vi "SUB-Excel-Function-SLOPE.vi"(10 "Y":dbl[](array[numeric]), 11 "X":dbl[](array[numeric])) -> (1 "offset":dbl, 2 "intercept":dbl format="%#.6g", 3 "slope":dbl format="%#.6g")   [LabVIEW 2015]
uses:
  <vilib>/Analysis/baseanly.llb/Mean (DBL).vi
  <vilib>/Analysis/NI_AALBase.lvlib
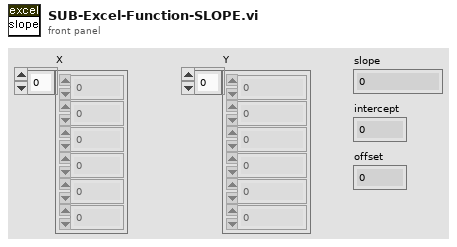
[diagram p1: front panel]
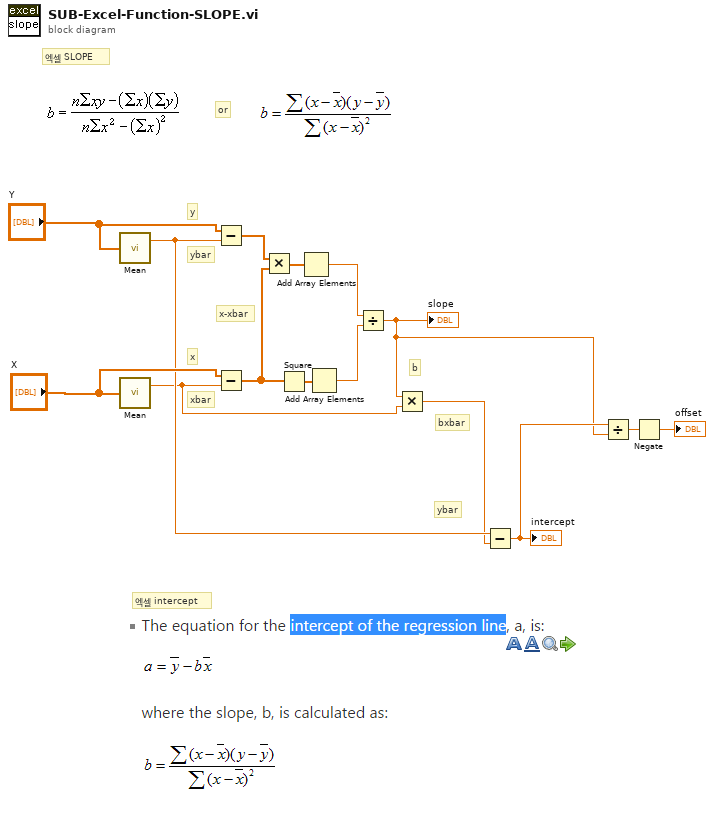
[diagram p0: block diagram]
diagram:
  # "bxbar"
  # "b"
  # "ybar"
  # "엑셀 intercept"
  # "x-xbar"
  # "y"
  # "ybar"
  # "x"
  # "xbar"
  # "or"
  # "엑셀 SLOPE"
  n1 = call-poly <vilib>:"Mean.vi"("X"="Y") -> ("mean"=w7:dbl)  [unwired: 1 out]
  n2 = call-poly <vilib>:"Mean.vi"("X"="X") -> ("mean"=w6:dbl)  [unwired: 1 out]
  n3 = Subtract(x="Y", y=w7) -> (x-y=w12:dbl[])
  n4 = Subtract(x="X", y=w6) -> (x-y=w10:dbl[])
  n5 = Multiply(x=w12, y=w10) -> (x*y=w9:dbl[])
  n6 = Square(x=w10) -> (x^2=w11:dbl[])
  n7 = Add Array Elements(numeric array=w9) -> (sum=w8:dbl)
  n8 = Add Array Elements(numeric array=w11) -> (sum=w13:dbl)
  n9 = Divide(x=w8, y=w13) -> (x/y=w3:dbl)
  "slope" <- w3
  n10 = Multiply(x=w3, y=w6) -> (x*y=w5:dbl)
  n11 = Subtract(x=w7, y=w5) -> (x-y=w4:dbl)
  "intercept" <- w4
  n12 = Divide(x=w4, y=w3) -> (x/y=w2:dbl)
  n13 = Negate(x=w2) -> (-x=→"offset":dbl)
